vi "InterpetOffset (SubVI).vi"(9 "Y offset":sgl, 10 "X offset":sgl, 11 "Good position":bool) -> (3 "Offset interpreter":T1)   [LabVIEW 2016]
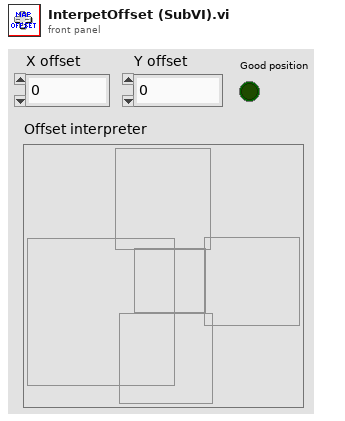
[diagram p1: front panel]
types:
  T1 = cluster{"Offset Interpreter - Right":bool, "Offset Interpreter - forward":bool, "Offset Interpreter - backward":bool, "Offset Interpreter - Left":bool, "Placement Confirmation":bool}
  T2 = cluster{"Offset Interpreter - Right":bool, "Offset Interpreter - Down":bool, "Offset Interpreter - Up":bool, "Offset Interpreter - Left":bool, "Placement Confirmation":bool}
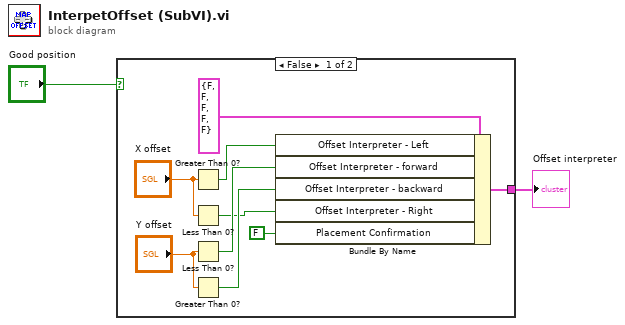
[diagram p0: block diagram]
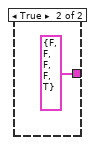
[diagram p2: hidden frame]
diagram:
  n1 = case shown="False" "Good position" {
    tunnel: [w10 T2 {"Offset Interpreter - Right"=FALSE, "Offset Interpreter - Down"=FALSE, "Offset Interpreter - Up"=FALSE, "Offset Interpreter - Left"=FALSE, "Placement Confirmation"=TRUE} ("Offset interpreter")] -> w1
    frame False {
      n2 = Greater Than 0?(x="X offset") -> (x > 0?=w3:bool)
      n3 = Less Than 0?(x="X offset") -> (x < 0?=w4:bool)
      n4 = Less Than 0?(x="Y offset") -> (x < 0?=w5:bool)
      n5 = Greater Than 0?(x="Y offset") -> (x > 0?=w6:bool)
      n6 = Bundle By Name(cluster=T1 {"Offset Interpreter - Right"=FALSE, "Offset Interpreter - forward"=FALSE, "Offset Interpreter - backward"=FALSE, "Offset Interpreter - Left"=FALSE, "Placement Confirmation"=FALSE} ("Offset interpreter"), "Offset Interpreter - Left"=w3, "Offset Interpreter - forward"=w5, "Offset Interpreter - backward"=w6, "Offset Interpreter - Right"=w4, "Placement Confirmation"=FALSE) -> (w10:T1)
    }
    frame True {
    }
  }
  "Offset interpreter" <- w1
